vi "Disconncetion DB.vi"(8 "error in (no error)":errorcluster caption="错误输入（无错误）", 11 "Connncet State":T1) -> (0 "error out":errorcluster caption="错误输出", 3 "Connect State":T1)   [LabVIEW 2014]
uses:
  <vilib>/addons/database/NI_Database_API.lvlib
  <vilib>/addons/database/Connection.llb/Conn ObjectReference.ctl
  Ctr/Constr.ctl
  Ctr/Conneect State.ctl
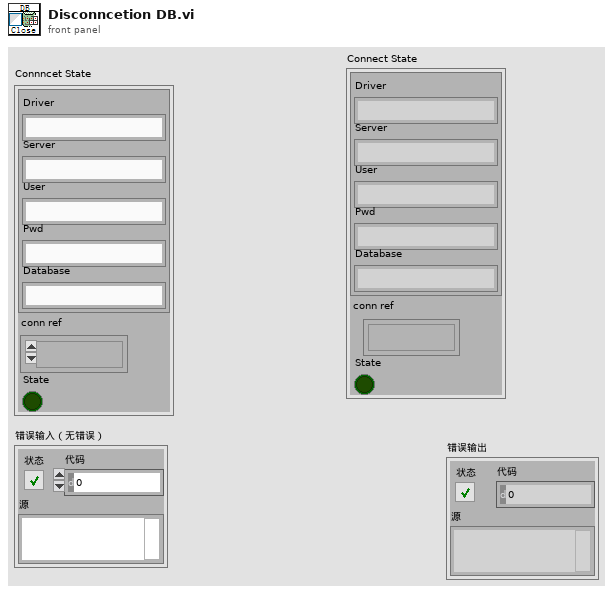
[diagram p1: front panel]
types:
  T1 = typedef "Conneect State.ctl" = cluster{"Constr":T2, "conn ref":T3, "State":bool}
  T2 = typedef "Constr.ctl" = cluster{"Driver":string, "Server":string, "User":string, "Pwd":string, "Database":string}
  T3 = typedef "NI_Database_API.lvlib/Conn ObjectReference.ctl" = refnum<k1>
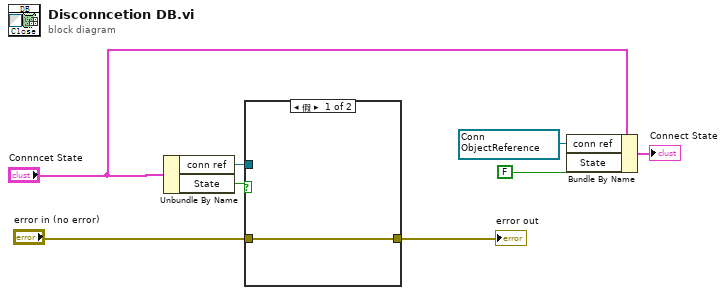
[diagram p0: block diagram]
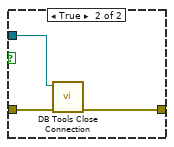
[diagram p2: hidden frame]
diagram:
  w5 = T3 refnum items=["Connection"] ("conn ref")
  n1 = Unbundle By Name("Connncet State") -> ("conn ref"=w1:T3, "State"=w2:bool)
  n2 = case shown="假" w2 {
    tunnel: "error in (no error)" -> [w9 w12]
    tunnel: w1 -> [_ w11]
    tunnel: [w9 w10] -> w7
    frame False {
    }
    frame True {
      n3 = call <vilib>:"DB Tools Close Connection.vi"("error in (no error)"=w12, "connection reference"=w11) -> ("error out"=w10:errorcluster)  [unwired: 5 in]
    }
  }
  "error out" <- w7
  n4 = Bundle By Name(cluster="Connncet State", "conn ref"=w5, "State"=FALSE) -> (→"Connect State":T1)
